vi "Log_CleanUp.vi"(8 "error in (no error)":errorcluster) -> (0 "error out":errorcluster)   [LabVIEW 2023, in "Log.lvclass"]
uses:
  Log.lvclass
  Log_Facility.ctl
  Log_Level.ctl
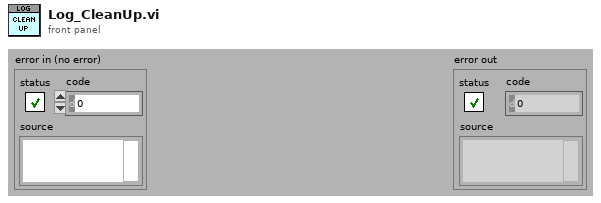
[diagram p1: front panel]
types:
  T1 = typedef "Log.lvclass/ObjectAttributes.ctl" = cluster{"Level":T2, "Facilities":variant, "Event":refnum<user-event>}
  T2 = typedef "Log.lvclass/Log_Level.ctl" = enum16{"none", "info", "trace", "warn", "error", "fatal"}
  T3 = typedef "Log.lvclass/Log_Facility.ctl" = cluster{"Path":path, "Ref":refnum<file>, "Level":T2}
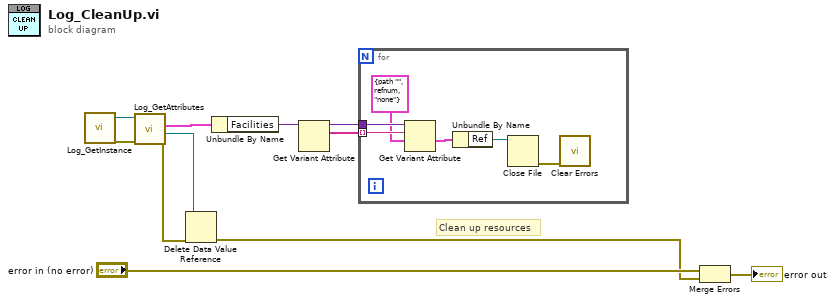
[diagram p0: block diagram]
diagram:
  # "Clean up resources"
  n1 = call "Log_GetInstance.vi"() -> ("error out"=w9:errorcluster, "reference out"=w8:refnum<class "Log.lvclass">)  [unwired: 7 in, 3 out]
  n2 = call "Log_GetAttributes.vi"("error in (no error)"=w9, "reference in"=w8) -> ("error out"=w7:errorcluster, "DataRef"=w6:refnum<data-value>, "Data"=w10:T1)  [unwired: 6 in, 1 out]
  n3 = Delete Data Value Reference(data value reference=w6, error in=w7) -> (error out=w1:errorcluster)  [unwired: 1 out]
  n4 = Unbundle By Name(w10) -> ("Facilities"=w4:variant)
  n5 = Get Variant Attribute(Variant=w4) -> (duplicate Variant=w3:variant, names=w2:string[])  [unwired: 3 in, 2 out]
  n6 = for {
    tunnel: w3 -> [w17]
    tunnel: w2 -> [w16] mode=indexing
    n7 = Get Variant Attribute(Variant=w17, name=w16, default value (empty Variant)=T3 {"Path"=path "", "Ref"=refnum, "Level"=enum."none"} ("Cluster")) -> (value=w14:T3)  [unwired: 1 in, 3 out]
    n8 = Unbundle By Name(w14) -> ("Ref"=w13:refnum<file>)
    n9 = Close File(refnum=w13) -> (error out=w12:errorcluster)  [unwired: 1 in, 1 out]
    n10 = call <vilib>:"Clear Errors.vi"("error in (no error)"=w12) -> ()  [unwired: 5 in, 2 out]
  }
  n11 = Merge Errors("error in (no error)", w1) -> (→"error out":errorcluster)
